vi "MainApp.vi"() -> ()   [LabVIEW 2018]
uses:
  TyDefApp/StatesApp.ctl
  TypeDefSERVER/PersonaFisica.ctl
  TypeDefSERVER/PersonaMoral.ctl
  TypeDefSERVER/ID_REQUEST.ctl
  <vilib>/httpClient/PUTBuffer.vi
  <vilib>/Utility/config.llb/Read Key (String).vi
  <vilib>/Utility/config.llb/Write Key (String).vi
  <vilib>/httpClient/LabVIEWHTTPClient.lvlib
  <vilib>/Utility/config.llb/NI_LVConfig.lvlib
panel:
  in  "MenuOpciones":enum32{"MenuPrincipal", "MenuCreditoPyme"}(tab)
  in  "SolicitudesRecientes_btn":bool
  in  "CreditoPyme_btn":bool
  out "CreditoPyme_select":bool
  out "SolicitudesRecientes_select":bool
  in  "PersonaFisica_btn":bool
  in  "PersonaMoral_btn":bool
  out "PersonaMoral_select":bool
  out "PersonaFisica_select":bool
  in  "PaginasPrincipales":T1(tab)
  in  "NoTengoCuenta_btn":bool
  in  "SoyCliente_btn":bool
  in  "SolicitudesRecientes_table":i32(listbox)
  in  "FinalizarSolicitud_btn":bool
  in  "IrADatosEspecificos_btn":bool caption="Siguiente:"
  in  "inicio_btn":bool
  in  "MenuPersonaFisica_Moral":T2(tab)
  in  "¿Para que es el credito?":string
  in  "Años de tu negocio:":i32
  in  "Sector de tu negocio:":string
  in  "Correo:":string
  in  "Celular (10 digitos):":string
  in  "RFC con homoclave:":string
  in  "Apellido paterno:":string
  in  "Apellido materno:":string
  in  "Nombre:":string
  in  "Correo_Moral":string caption="Correo:"
  in  "Celular_Moral":string caption="Celular (10 digitos):"
  in  "ApellidoPaterno_Moral":string caption="Apellido paterno:"
  in  "ApellidoMaterno_Moral":string caption="Apellido materno:"
  in  "Nombre_Moral":string caption="Nombre:"
  in  "Moral1_btn":bool
  in  "RazonSocial":string caption="Razon social:"
  in  "RFC_Moral":string caption="RFC con homoclave:"
  in  "SectorDeNegocio_Moral2":string caption="Sector de tu negocio:"
  in  "AñosDenegocio_Moral2":i32 caption="Años de tu negocio:"
  in  "ParaQueCredito_Moral2":string caption="¿Para que es el credito?"
  in  "Moral2_btn":bool caption="Back Tool"
  in  "Garantia, patrimonio (valor):":dbl format="$%#_g"
  in  "Numero de empleados:":i32
  in  "Numero de sucursales:":i32
  in  "Regimen que tributa:":string
  in  "Años de antiguedad de la empresa:":i32
  in  "Flujo de efectivo mensual:":dbl format="$%#_g"
  in  "Utilidad neta:":dbl format="$%#_g"
  in  "Capital social:":dbl format="$%#_g"
  in  "Importe Total:":dbl format="$%#_g"
  # "Solicita tu credito Pyme aqui."
  # "Solicitud de credito para cliente BBVA"
  # "Datos del presentante legal:"
  # "Datos del negocio"
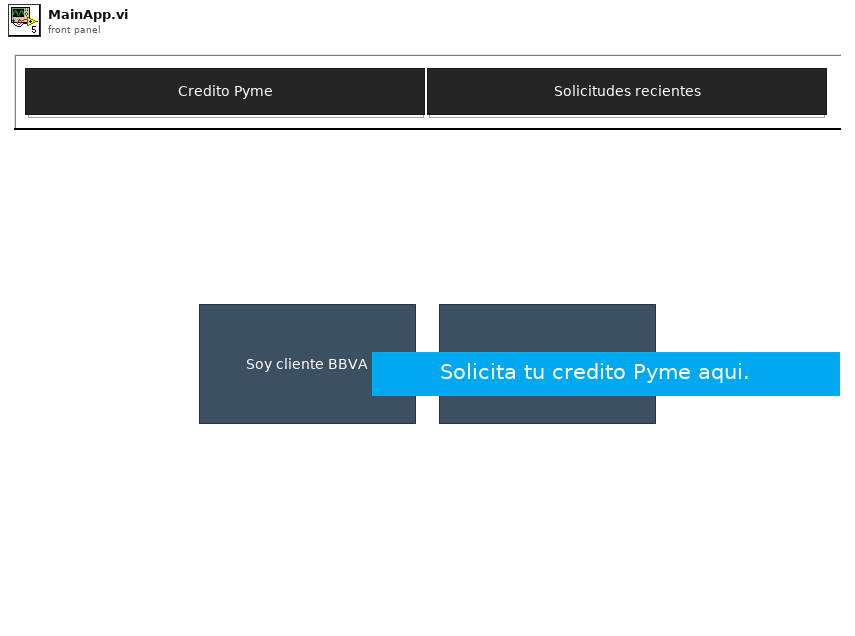
[diagram p1: front panel]
types:
  T1 = enum32{"CreditoPyme", "SolicitudesRecientes", "PersonaFisica", "PersonaMoral", "None", "DatosEspecificos"}
  T2 = enum32{"PersonaFisica", "PersonaMoral1", "PersonaMoral 2", "DatosEspecificos"}
  T3 = enum16{"init", "standBy", "goToCreditoPyme", "goToSolicitudesRecientes", "goToPersonaFisica", "goToPersonaMoral1", "goToPersonaMoral2", "goToDatosEspecificos", "ClearEntrys", "DeleteHistorial", "ShowSolicitudAceptada", "ShowSolicitudCancelada", "RegisterSolicitudToCheck", "CloseApp"}
  T4 = typedef "StatesApp.ctl" = cluster{"Machine":enum16{"StateMachine", "Queues"}, "States":enum16{"init", "standBy", "goToCreditoPyme", "goToSolicitudesRecientes", "goToPersonaFisica", "goToPersonaMoral1", "goToPersonaMoral2", "goToDatosEspecificos", "ClearEntrys", "DeleteHistorial", "ShowSolicitudAceptada", "ShowSolicitudCancelada", "RegisterSolicitudToCheck", "CloseApp", "goToPersonaMoral", "CheckIsClient"}, "URL":string, "TipoPersona":string, "EsCliente?":bool, "ID_CARD":string}
  T5 = enum32{"Invalid", "Standard", "Closed", "Hidden", "Minimized", "Maximized"}
  T6 = typedef "NI_LVConfig.lvlib/Config Data RefNum.ctl" = refnum<k1>
  T7 = typedef "PersonaFisica.ctl" = cluster{"Sector de tu negocio":string, "Para que es el credito":string, "Correo":string, "RFC con homoclave":string, "Nombre":string, "Celular":string, "Apellido materno":string, "Apellido paterno":string, "Años de tu negocio:":i32, "Numero de tarjeta":string, "EsCliente?":bool, "Importe Total":dbl, "Capital social":dbl, "Flujo de efectivo mensual":dbl, "Utilidad neta":dbl, "Garantia, patrimonio (valor):":dbl, "Numero de sucursales":i32, "Numero de empleados":i32, "Años de antiguedad de la empresa":i32, "Regimen que tributa":string, "Confirmado?":bool, "TipoPersona":string}
  T8 = typedef "PersonaMoral.ctl" = cluster{"Sector del negocio":string, "Para que el credito":string, "RFC":string, "RazonSocial":string, "Apellido paterno":string, "Nombre":string, "Correo":string, "Apellido materno":string, "Celular":string, "AñosDenegocio":i32, "Numero de tarjeta":string, "EsCliente?":bool, "Importe Total":dbl, "Capital social":dbl, "Flujo de efectivo mensual":dbl, "Utilidad neta":dbl, "Garantia, patrimonio (valor):":dbl, "Numero de sucursales":i32, "Numero de empleados":i32, "Años de antiguedad de la empresa":i32, "Regimen que tributa":string, "Confirmado?":bool, "TipoPersona":string}
  T9 = enum16{"CreditoPyme", "SolicitudeRecientes", "PersonaFisica", "PersonaMoral"}
  T10 = enum16{"init", "standBy", "goToCreditoPyme", "goToSolicitudesRecientes", "goToPersonaFisica", "goToPersonaMoral1", "goToPersonaMoral2", "goToDatosEspecificos", "ClearEntrys", "DeleteHistorial", "ShowSolicitudAceptada", "ShowSolicitudCancelada", "RegisterSolicitudToCheck", "CloseApp", "goToPersonaMoral"}
  T11 = enum32{"PersonaFisica", "PersonaMoral1", "PersonaMoral 2"}
  T12 = enum16{"init", "standBy", "goToCreditoPyme", "goToSolicitudesRecientes", "goToPersonaFisica", "goToPersonaMoral1", "goToPersonaMoral2", "goToDatosEspecificos", "ClearEntrys", "DeleteHistorial", "ShowSolicitudAceptada", "ShowSolicitudCancelada", "RegisterSolicitudToCheck", "CloseApp", "goToPersonaMoral", "CheckIsClient"}
  T13 = typedef "ID_REQUEST.ctl" = cluster{"ID":i32[]}
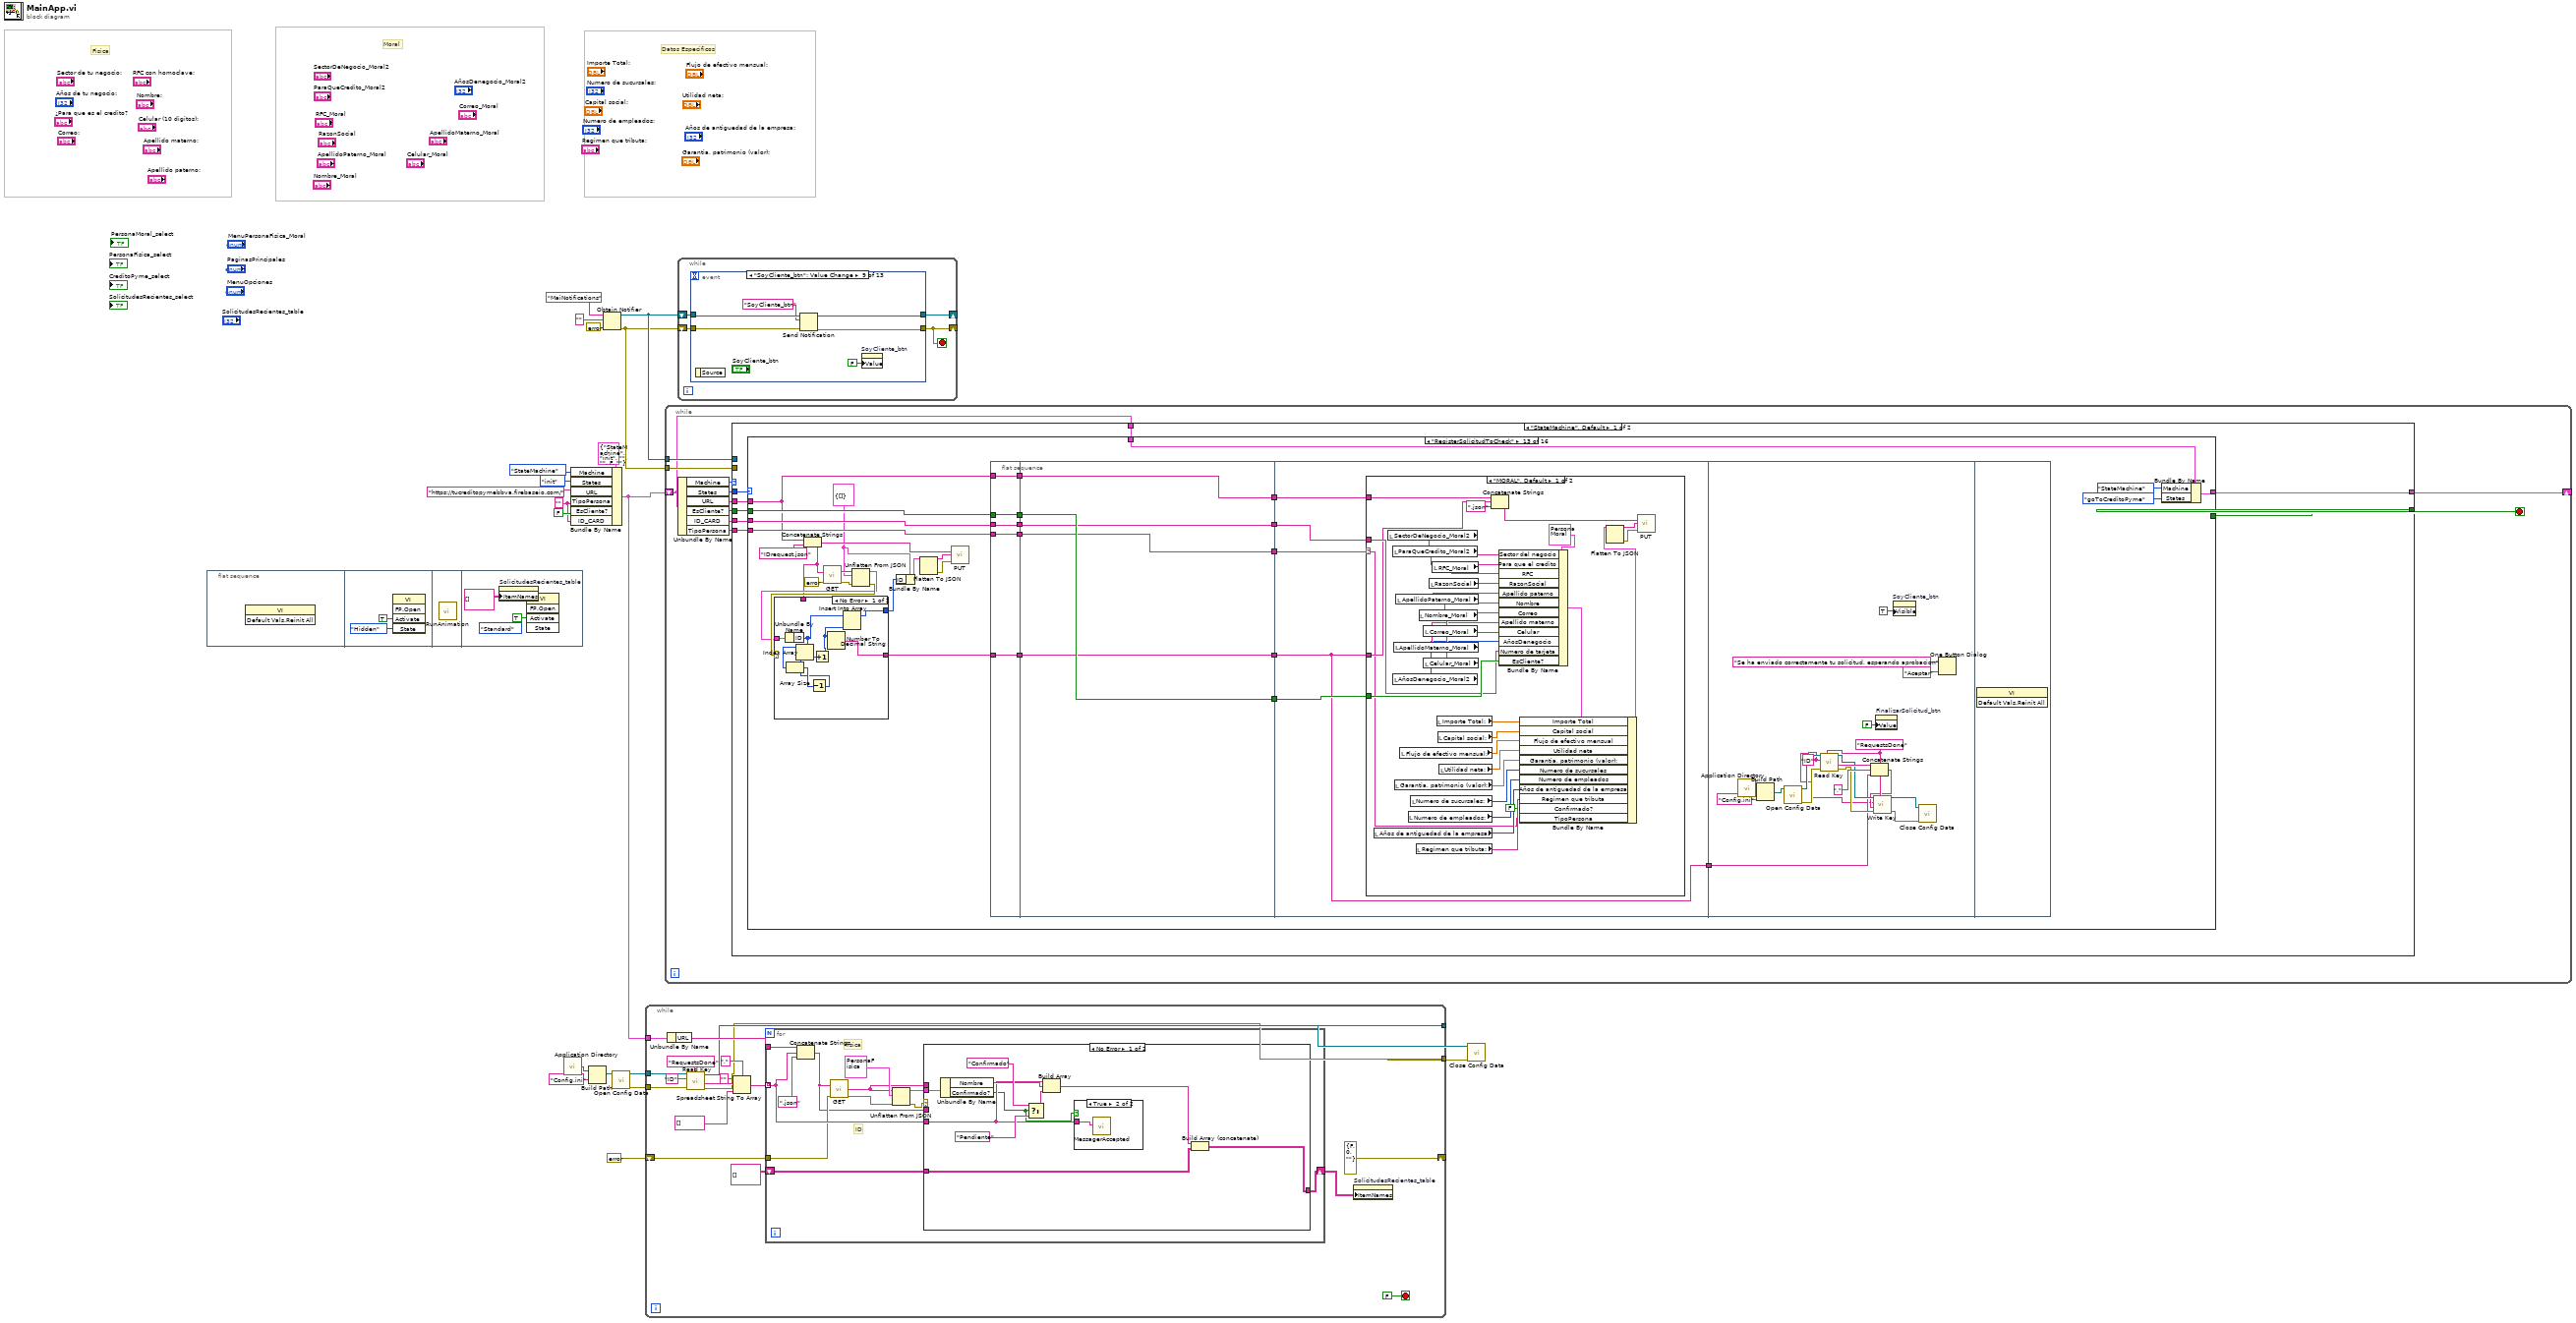
[diagram p0: block diagram]
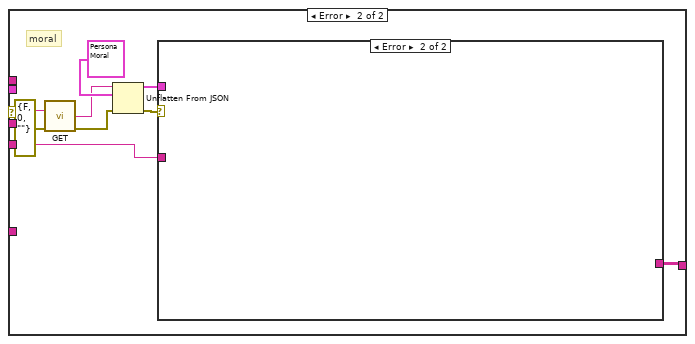
[diagram p3: hidden frame]
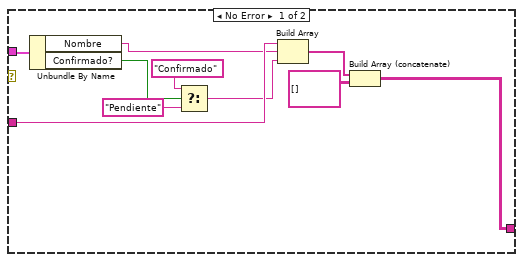
[diagram p4: hidden frame]
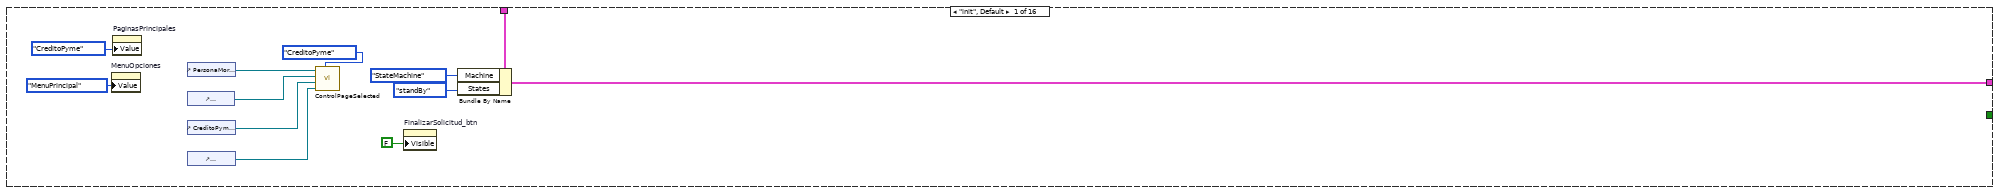
[diagram p5: hidden frame]
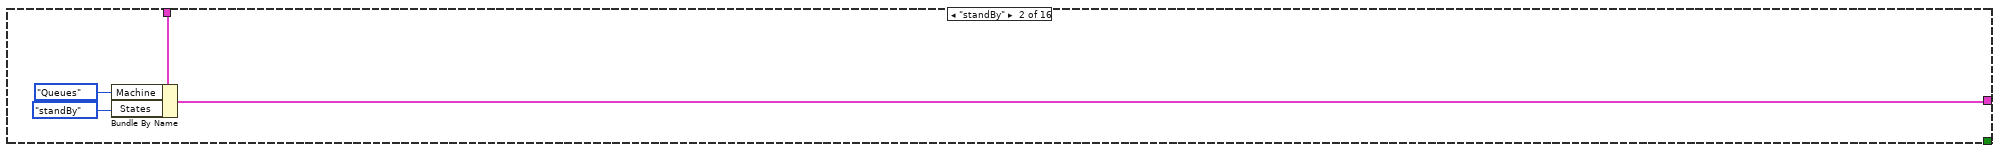
[diagram p6: hidden frame]
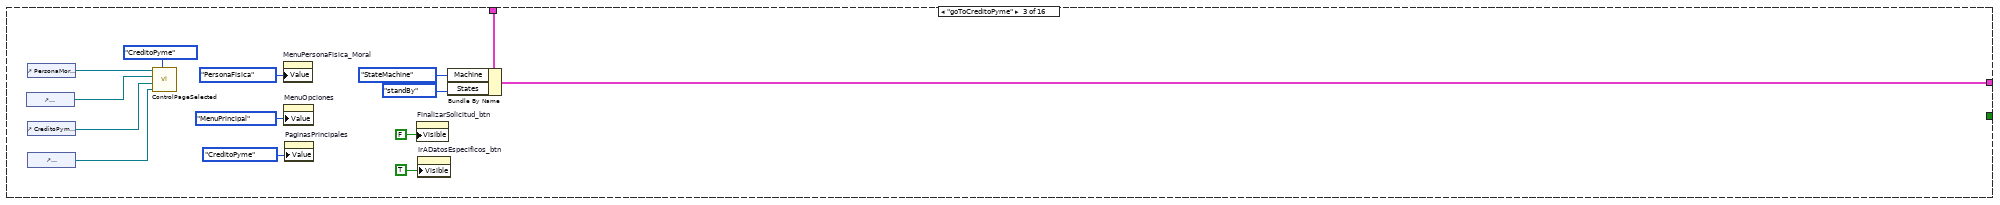
[diagram p7: hidden frame]
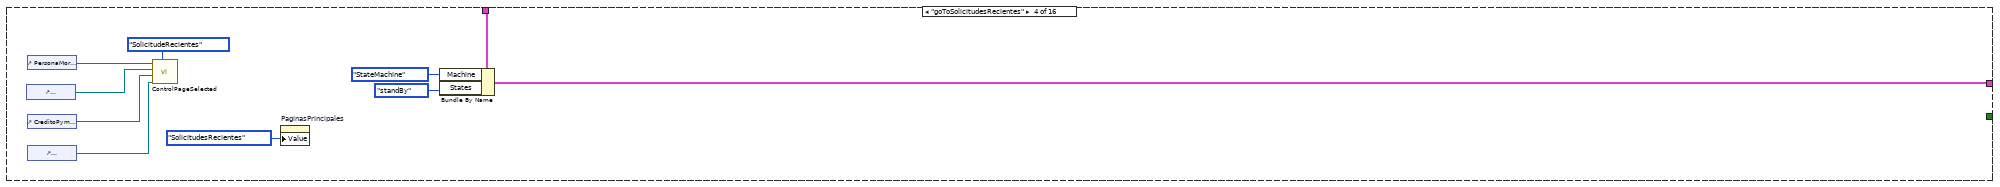
[diagram p8: hidden frame]
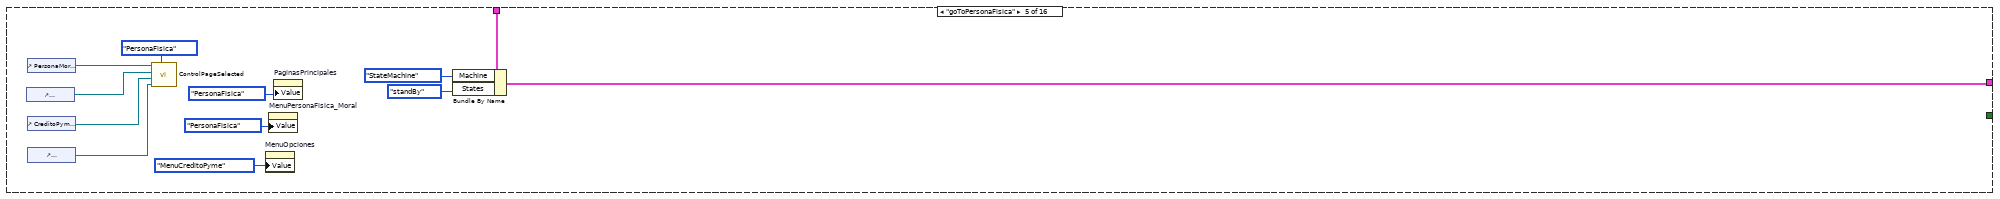
[diagram p9: hidden frame]
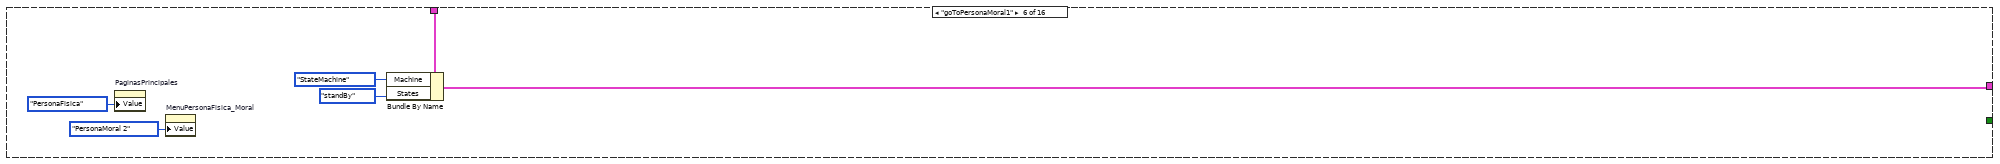
[diagram p10: hidden frame]
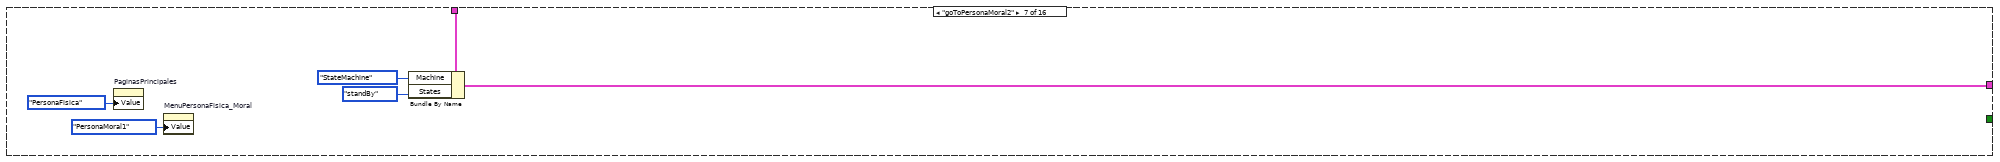
[diagram p11: hidden frame]
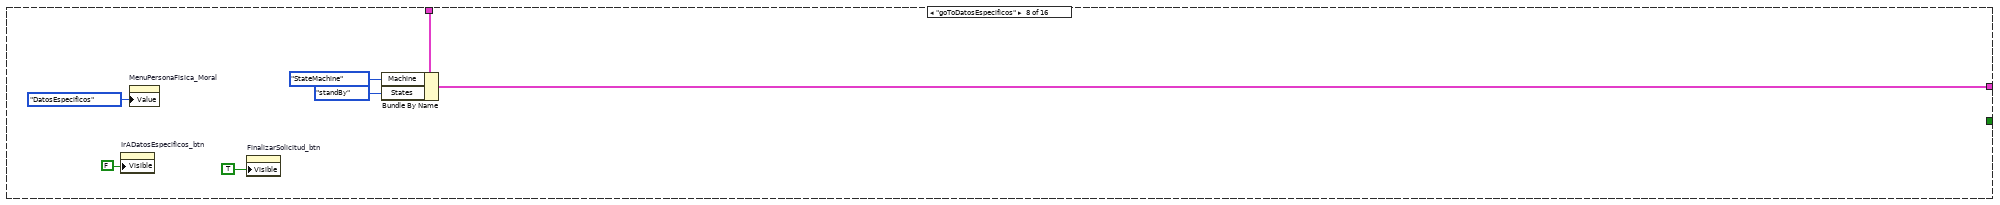
[diagram p12: hidden frame]
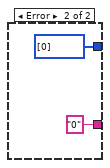
[diagram p17: hidden frame]
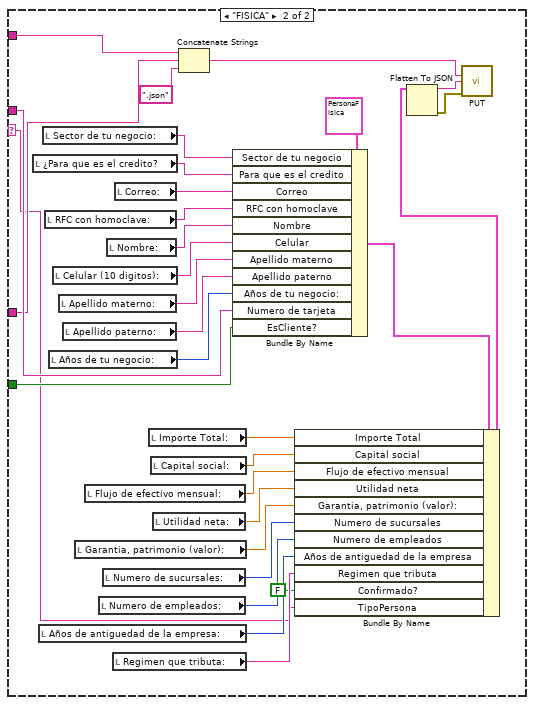
[diagram p18: hidden frame]
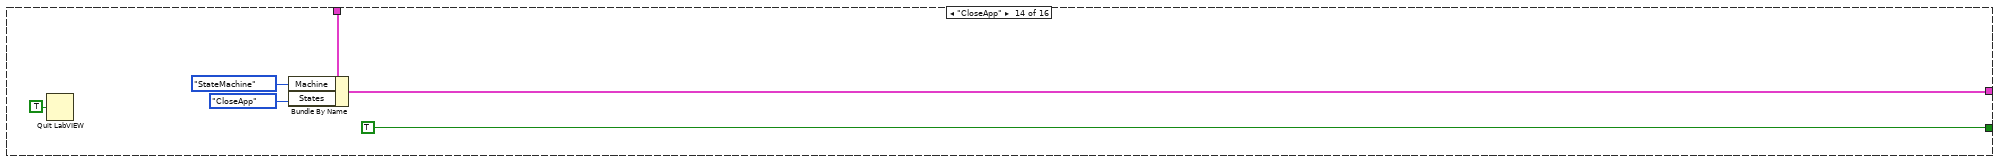
[diagram p19: hidden frame]
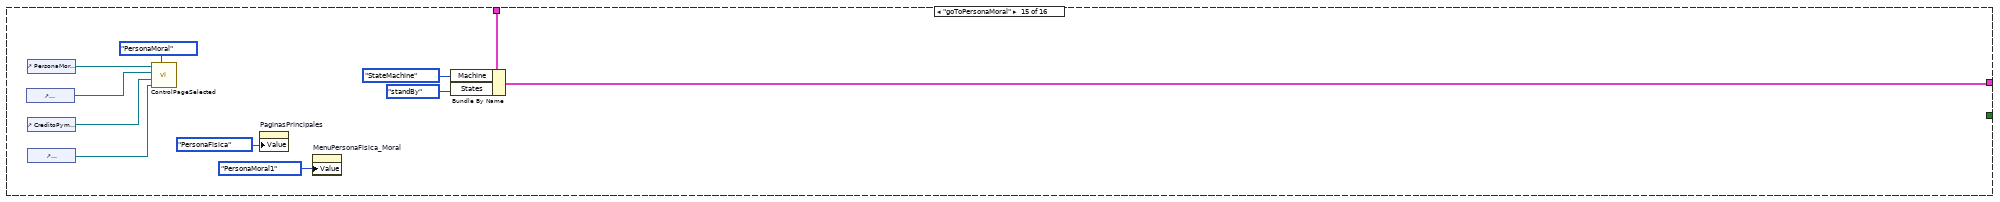
[diagram p20: hidden frame]
diagram:
  w10 = "" ("TipoPersona")
  # "Datos Especificos"
  # "Moral"
  # "Fisica"
  n1 = flat-sequence {
    frame #0 {
      n2 = invoke class="VI" method="Default Vals.Reinit All"() -> ()  [unwired: 3 in, 3 out]
    }
    frame #1 {
      n3 = invoke class="VI" method="FP.Open"("Activate"=TRUE ("Activate?"), "State"=T5."Hidden") -> ()  [unwired: 3 in, 5 out]
    }
    frame #2 {
      n4 = call "RunAnimation.vi"() -> ()  [unwired: 12 in]
    }
    frame #3 {
      (unwired) T5."Standard" ("State")
      n5 = property on="SolicitudesRecientes_table" class="MCListbox (strict)"("ItemNames"=string[][] [] ("Item Names")) -> ()  [unwired: 2 in, 2 out]
      n6 = invoke class="VI" method="FP.Open"("Activate"=TRUE ("Activate?")) -> ()  [unwired: 4 in, 5 out]
    }
  }
  n7 = call <vilib>:"Application Directory.vi"() -> ("Application Directory"=w7:path)
  n8 = Bundle By Name(cluster=T4 {"Machine"=enum."StateMachine", "States"=enum."init", "URL"="", "TipoPersona"="", "EsCliente?"=FALSE, "ID_CARD"=""} ("Cluster"), "Machine"=enum16{"StateMachine", "Queues"}."StateMachine", "States"=T3."init", "URL"="https://tucreditopymebbva.firebaseio.com/", "TipoPersona"=w10, "EsCliente?"=FALSE, "ID_CARD"=w10) -> (w4:T4)
  n9 = Build Path(base path=w7, name or relative path="Config.ini") -> (appended path=w5:path)
  n10 = Obtain Notifier(name (unnamed)="MaiNotifications", notification data type="", error in (no error)=errorcluster {"status"=FALSE, "code"=0, "source"=""}) -> (notifier out=w16:refnum<notifier>, error out=w15:errorcluster)  [unwired: 1 in, 1 out]
  n11 = call <vilib>:"Open Config Data.vi"("configuration file path"=w5) -> ("error out"=w8:errorcluster, "refnum"=w9:T6)  [unwired: 8 in, 1 out]
  n12 = while {
    tunnel: w9 -> [w41]
    tunnel: w8 -> [w40]
    tunnel: w4 -> [w33]
    tunnel: [w31] -> w3
    tunnel: [w30] -> w2
    shift-right: [errorcluster {"status"=FALSE, "code"=0, "source"=""} ("error in (no error)")] -> _
    shift-left: errorcluster {"status"=FALSE, "code"=0, "source"=""} ("error in (no error)") -> [w28]
    stop <- FALSE stop-if-true
    n13 = Unbundle By Name(w33) -> ("URL"=w32:string)
    n14 = call-poly <vilib>:"Read Key.vi"("section"="RequestsDone", "error in (no error)"=w40, "key"="ID", "refnum"=w41) -> ("error out"=w30:errorcluster, "value"=w37:string, "refnum out"=w31:T6)  [unwired: 4 in, 1 out]
    n15 = Spreadsheet String To Array(delimiter (Tab)=",", format string="", spreadsheet string=w37, array type (2D Dbl)=string[] []) -> (array=w34:string[])
    n16 = for {
      tunnel: w34 -> [w48] mode=indexing
      tunnel: w32 -> [w54]
      tunnel: w28 -> [w46]
      shift-right: [w44] -> w26
      shift-left: string[][] [] -> [w43]
      # "ID"
      # "fisica"
      n17 = Concatenate Strings(w54, w48, ".json" ("string")) -> (w45:string)
      n18 = call <vilib>:"GET.vi"("url"=w45, "error in (no error)"=w46) -> ("body"=w47:string, "error out"=w52:errorcluster)  [unwired: 10 in, 2 out]
      n19 = Unflatten From JSON(JSON string=w47, type and defaults=T7 {"Sector de tu negocio"="", "Para que es el credito"="", "Correo"="", "RFC con homoclave"="", "Nombre"="", "Celular"="", "Apellido materno"="", "Apellido paterno"="", "Años de tu negocio:"=0, "Numero de tarjeta"="", "EsCliente?"=FALSE, "Importe Total"=0.0, "Capital social"=0.0, "Flujo de efectivo mensual"=0.0, "Utilidad neta"=0.0, "Garantia, patrimonio (valor):"=0.0, "Numero de sucursales"=0, "Numero de empleados"=0, "Años de antiguedad de la empresa"=0, "Regimen que tributa"="", "Confirmado?"=FALSE, "TipoPersona"=""} ("Cluster"), error in (no error)=w52) -> (value=w49:T7, error out=w50:errorcluster)  [unwired: 4 in]
      n20 = case shown="No Error" w50 {
        tunnel: w49 -> [w64 _]
        tunnel: w47 -> [_ _]
        tunnel: w48 -> [w57 w71]
        tunnel: [w59 w70] -> w44
        tunnel: w45 -> [_ w67]
        tunnel: w43 -> [w58 _]
        frame No Error {
          n21 = Unbundle By Name(w64) -> ("Nombre"=w61:string, "Confirmado?"=w55:bool)
          n22 = Select(t="Confirmado", s=w55, f="Pendiente") -> (s? t:f=w56:string)
          n23 = Build Array(w57, w61, w56) -> (w60:string[])
          n24 = case shown="True" w55 {
            tunnel: w57 -> [_ w65]
            frame False {
            }
            frame True {
              n25 = call "MessagerAccepted.vi"("id"=w65) -> ()  [unwired: 11 in]
            }
          }
          n26 = Build Array (concatenate)(w60, w58) -> (w59:string[][])
        }
        frame Error {
          # "moral"
          n27 = call <vilib>:"GET.vi"("url"=w67, "error in (no error)"=errorcluster {"status"=FALSE, "code"=0, "source"=""}) -> ("body"=w68:string, "error out"=w69:errorcluster)  [unwired: 10 in, 2 out]
          n28 = Unflatten From JSON(JSON string=w68, type and defaults=T8 {"Sector del negocio"="", "Para que el credito"="", "RFC"="", "RazonSocial"="", "Apellido paterno"="", "Nombre"="", "Correo"="", "Apellido materno"="", "Celular"="", "AñosDenegocio"=0, "Numero de tarjeta"="", "EsCliente?"=FALSE, "Importe Total"=0.0, "Capital social"=0.0, "Flujo de efectivo mensual"=0.0, "Utilidad neta"=0.0, "Garantia, patrimonio (valor):"=0.0, "Numero de sucursales"=0, "Numero de empleados"=0, "Años de antiguedad de la empresa"=0, "Regimen que tributa"="", "Confirmado?"=FALSE, "TipoPersona"=""} ("Cluster"), error in (no error)=w69) -> (value=w72:T8, error out=w73:errorcluster)  [unwired: 4 in]
          n29 = case shown="Error" w73 {
            tunnel: w72 -> [w84 _]
            tunnel: w71 -> [w80 _]
            tunnel: [w75 _] -> w70
            frame No Error {
              n30 = Unbundle By Name(w84) -> ("Nombre"=w79:string, "Confirmado?"=w83:bool)
              n31 = Select(t="Confirmado", s=w83, f="Pendiente") -> (s? t:f=w78:string)
              n32 = Build Array(w80, w79, w78) -> (w77:string[])
              n33 = Build Array (concatenate)(w77, string[][] [] ("element")) -> (w75:string[][])
            }
            frame Error {
            }
          }
        }
      }
    }
    n34 = property on="SolicitudesRecientes_table" class="MCListbox (strict)"("ItemNames"=w26) -> ()  [unwired: 2 in, 2 out]
  }
  n35 = while {
    shift-right: [w89] -> _
    shift-left: w4 -> [w90]
    tunnel: w16 -> [w92]
    tunnel: w15 -> [w91]
    stop <- w88 stop-if-true
    n36 = Unbundle By Name(w90) -> ("Machine"=w95:enum16{"StateMachine", "Queues"}, "States"=w94:T12, "URL"=w93:string, "EsCliente?"=w87:bool, "ID_CARD"=w86:string, "TipoPersona"=w85:string)
    n37 = case shown="\"StateMachine\", Default" w95 {
      tunnel: w94 -> [w103 _]
      tunnel: w93 -> [w102 _]
      tunnel: w92 -> [_ w347]
      tunnel: w91 -> [_ w346]
      tunnel: w90 -> [w98 w344]
      tunnel: [w101 w343] -> w89
      tunnel: [w100 _] -> w88
      tunnel: w87 -> [w99 _]
      tunnel: w86 -> [w97 _]
      tunnel: w85 -> [w96 _]
      frame "StateMachine", Default {
        n38 = case shown="\"RegisterSolicitudToCheck\"" w103 {
          tunnel: w102 -> [_ _ _ _ _ _ _ _ _ _ _ _ w191 _ _ _]
          tunnel: w98 -> [w113 w119 w133 w141 w153 w159 w165 w174 _ _ _ _ w206 w317 w328 w333]
          tunnel: [w112 w118 w132 w140 w152 w158 w164 w173 _ _ _ _ w205 w316 w327 w332] -> w101
          tunnel: [_ _ _ _ _ _ _ _ _ _ _ _ _ TRUE _ _] -> w100
          tunnel: w99 -> [_ _ _ _ _ _ _ _ _ _ _ _ w201 _ _ w334]
          tunnel: w97 -> [_ _ _ _ _ _ _ _ _ _ _ _ w200 _ _ _]
          tunnel: w96 -> [_ _ _ _ _ _ _ _ _ _ _ _ w202 _ _ _]
          frame "init", Default {
            n39 = property on="MenuOpciones" class="TabCtl (strict)"("Value"=enum32{"MenuPrincipal", "MenuCreditoPyme"}."MenuPrincipal" ("MenuOpciones")) -> ()  [unwired: 2 in, 2 out]
            n40 = property on="PaginasPrincipales" class="TabCtl (strict)"("Value"=T1."CreditoPyme" ("PaginasPrincipales")) -> ()  [unwired: 2 in, 2 out]
            n41 = control-ref of="PersonaFisica_select"() -> (w109:refnum<vi>)
            n42 = control-ref of="PersonaMoral_select"() -> (w110:refnum<vi>)
            n43 = control-ref of="CreditoPyme_select"() -> (w108:refnum<vi>)
            n44 = control-ref of="SolicitudesRecientes_select"() -> (w107:refnum<vi>)
            n45 = call "ControlPageSelected.vi"("PageSelected"=T9."CreditoPyme", "SolicitudesRecientes"=w107, "CreditoPyme"=w108, "PersonaFisica"=w109, "PersonaMoral"=w110) -> ()  [unwired: 7 in]
            n46 = property on="FinalizarSolicitud_btn" class="Bool (strict)"("Visible"=FALSE) -> ()  [unwired: 2 in, 2 out]
            n47 = Bundle By Name(cluster=w113, "Machine"=enum16{"StateMachine", "Queues"}."StateMachine", "States"=T3."standBy") -> (w112:T4)
          }
          frame "standBy" {
            n48 = Bundle By Name(cluster=w119, "Machine"=enum16{"StateMachine", "Queues"}."Queues", "States"=T3."standBy") -> (w118:T4)
          }
          frame "goToCreditoPyme" {
            n49 = control-ref of="PersonaFisica_select"() -> (w128:refnum<vi>)
            n50 = control-ref of="PersonaMoral_select"() -> (w129:refnum<vi>)
            n51 = control-ref of="CreditoPyme_select"() -> (w127:refnum<vi>)
            n52 = control-ref of="SolicitudesRecientes_select"() -> (w126:refnum<vi>)
            n53 = call "ControlPageSelected.vi"("PageSelected"=T9."CreditoPyme", "SolicitudesRecientes"=w126, "CreditoPyme"=w127, "PersonaFisica"=w128, "PersonaMoral"=w129) -> ()  [unwired: 7 in]
            n54 = property on="MenuPersonaFisica_Moral" class="TabCtl (strict)"("Value"=T2."PersonaFisica" ("MenuPersonaFisica_Moral")) -> ()  [unwired: 2 in, 2 out]
            n55 = property on="MenuOpciones" class="TabCtl (strict)"("Value"=enum32{"MenuPrincipal", "MenuCreditoPyme"}."MenuPrincipal" ("MenuOpciones")) -> ()  [unwired: 2 in, 2 out]
            n56 = property on="PaginasPrincipales" class="TabCtl (strict)"("Value"=T1."CreditoPyme" ("PaginasPrincipales")) -> ()  [unwired: 2 in, 2 out]
            n57 = property on="FinalizarSolicitud_btn" class="Bool (strict)"("Visible"=FALSE ("FinalizarSolicitud_btn")) -> ()  [unwired: 2 in, 2 out]
            n58 = property on="IrADatosEspecificos_btn" class="Bool (strict)"("Visible"=TRUE) -> ()  [unwired: 2 in, 2 out]
            n59 = Bundle By Name(cluster=w133, "Machine"=enum16{"StateMachine", "Queues"}."StateMachine", "States"=T10."standBy") -> (w132:T4)
          }
          frame "goToSolicitudesRecientes" {
            n60 = control-ref of="PersonaFisica_select"() -> (w138:refnum<vi>)
            n61 = control-ref of="PersonaMoral_select"() -> (w139:refnum<vi>)
            n62 = control-ref of="CreditoPyme_select"() -> (w137:refnum<vi>)
            n63 = control-ref of="SolicitudesRecientes_select"() -> (w136:refnum<vi>)
            n64 = call "ControlPageSelected.vi"("PageSelected"=T9."SolicitudeRecientes", "SolicitudesRecientes"=w136, "CreditoPyme"=w137, "PersonaFisica"=w138, "PersonaMoral"=w139) -> ()  [unwired: 7 in]
            n65 = property on="PaginasPrincipales" class="TabCtl (strict)"("Value"=T1."SolicitudesRecientes" ("PaginasPrincipales")) -> ()  [unwired: 2 in, 2 out]
            n66 = Bundle By Name(cluster=w141, "Machine"=enum16{"StateMachine", "Queues"}."StateMachine", "States"=T10."standBy") -> (w140:T4)
          }
          frame "goToPersonaFisica" {
            n67 = control-ref of="PersonaFisica_select"() -> (w150:refnum<vi>)
            n68 = control-ref of="PersonaMoral_select"() -> (w151:refnum<vi>)
            n69 = control-ref of="CreditoPyme_select"() -> (w149:refnum<vi>)
            n70 = control-ref of="SolicitudesRecientes_select"() -> (w148:refnum<vi>)
            n71 = call "ControlPageSelected.vi"("PageSelected"=T9."PersonaFisica", "SolicitudesRecientes"=w148, "CreditoPyme"=w149, "PersonaFisica"=w150, "PersonaMoral"=w151) -> ()  [unwired: 7 in]
            n72 = property on="MenuOpciones" class="TabCtl (strict)"("Value"=enum32{"MenuPrincipal", "MenuCreditoPyme"}."MenuCreditoPyme" ("MenuOpciones")) -> ()  [unwired: 2 in, 2 out]
            n73 = property on="MenuPersonaFisica_Moral" class="TabCtl (strict)"("Value"=T11."PersonaFisica" ("MenuPersonaFisica_Moral")) -> ()  [unwired: 2 in, 2 out]
            n74 = property on="PaginasPrincipales" class="TabCtl (strict)"("Value"=T1."PersonaFisica" ("PaginasPrincipales")) -> ()  [unwired: 2 in, 2 out]
            n75 = Bundle By Name(cluster=w153, "Machine"=enum16{"StateMachine", "Queues"}."StateMachine", "States"=T10."standBy") -> (w152:T4)
          }
          frame "goToPersonaMoral1" {
            n76 = property on="PaginasPrincipales" class="TabCtl (strict)"("Value"=T1."PersonaFisica" ("PaginasPrincipales")) -> ()  [unwired: 2 in, 2 out]
            n77 = property on="MenuPersonaFisica_Moral" class="TabCtl (strict)"("Value"=T11."PersonaMoral 2" ("MenuPersonaFisica_Moral")) -> ()  [unwired: 2 in, 2 out]
            n78 = Bundle By Name(cluster=w159, "Machine"=enum16{"StateMachine", "Queues"}."StateMachine", "States"=T10."standBy") -> (w158:T4)
          }
          frame "goToPersonaMoral2" {
            n79 = property on="PaginasPrincipales" class="TabCtl (strict)"("Value"=T1."PersonaFisica" ("PaginasPrincipales")) -> ()  [unwired: 2 in, 2 out]
            n80 = property on="MenuPersonaFisica_Moral" class="TabCtl (strict)"("Value"=T11."PersonaMoral1" ("MenuPersonaFisica_Moral")) -> ()  [unwired: 2 in, 2 out]
            n81 = Bundle By Name(cluster=w165, "Machine"=enum16{"StateMachine", "Queues"}."StateMachine", "States"=T10."standBy") -> (w164:T4)
          }
          frame "goToDatosEspecificos" {
            n82 = property on="IrADatosEspecificos_btn" class="Bool (strict)"("Visible"=FALSE) -> ()  [unwired: 2 in, 2 out]
            n83 = property on="MenuPersonaFisica_Moral" class="TabCtl (strict)"("Value"=T2."DatosEspecificos" ("MenuPersonaFisica_Moral")) -> ()  [unwired: 2 in, 2 out]
            n84 = property on="FinalizarSolicitud_btn" class="Bool (strict)"("Visible"=TRUE ("FinalizarSolicitud_btn")) -> ()  [unwired: 2 in, 2 out]
            n85 = Bundle By Name(cluster=w174, "Machine"=enum16{"StateMachine", "Queues"}."StateMachine", "States"=T10."standBy") -> (w173:T4)
          }
          frame "ClearEntrys" {
          }
          frame "DeleteHistorial" {
          }
          frame "ShowSolicitudAceptada" {
          }
          frame "ShowSolicitudCancelada" {
          }
          frame "RegisterSolicitudToCheck" {
            w186 = T13 {"ID"=[]} ("Cluster")
            n86 = Concatenate Strings(w191, "IDrequest.json" ("string")) -> (w187:string)
            n87 = call <vilib>:"GET.vi"("url"=w187, "error in (no error)"=errorcluster {"status"=FALSE, "code"=0, "source"=""}) -> ("body"=w194:string, "error out"=w193:errorcluster)  [unwired: 10 in, 2 out]
            n88 = Unflatten From JSON(JSON string=w194, type and defaults=w186, error in (no error)=w193) -> (value=w188:T13, error out=w189:errorcluster)  [unwired: 4 in]
            n89 = case shown="No Error" w189 {
              tunnel: w188 -> [w214 _]
              tunnel: [w207 "0"] -> w181
              tunnel: w187 -> [_ _]
              tunnel: [w213 i32[] [0]] -> w185
              frame No Error {
                n90 = Unbundle By Name(w214) -> ("ID"=w212:i32[])
                n91 = Array Size(array=w212) -> (size(s)=w211:i32)
                n92 = Decrement(x=w211) -> (x-1=w210:i32)
                n93 = Index Array(array=w212, index=w210) -> (element=w209:i32)
                n94 = Increment(x=w209) -> (x+1=w208:i32)
                n95 = Number To Decimal String(number=w208) -> (decimal integer string=w207:string)  [unwired: 1 in]
                n96 = Insert Into Array(array=w212, new element=w208) -> (w213:i32[])  [unwired: 1 in]
              }
              frame Error {
              }
            }
            n97 = Bundle By Name(cluster=w186, "ID"=w185) -> (w184:T13)
            n98 = Flatten To JSON(anything=w184) -> (JSON string=w183:string, 11:w182:errorcluster)  [unwired: 2 in]
            n99 = call-poly <vilib>:"PUT.vi"("url"=w187, "buffer"=w183, "error in (no error)"=w182) -> ()  [unwired: 9 in, 4 out]
            n100 = flat-sequence {
              tunnel: w191 -> [w218]
              tunnel: w200 -> [w219]
              tunnel: w201 -> [w220]
              tunnel: w202 -> [w221]
              tunnel: [w221] -> w198
              tunnel: [w220] -> w197
              tunnel: [w219] -> w196
              tunnel: [w218] -> w195
              tunnel: w181 -> [w217]
              tunnel: [w217] -> w177
              tunnel: [w222] -> w199
              tunnel: w198 -> [w222]
              tunnel: w197 -> [w226]
              tunnel: w196 -> [w225]
              tunnel: w195 -> [w224]
              tunnel: [w226] -> w180
              tunnel: [w225] -> w179
              tunnel: [w224] -> w178
              tunnel: w177 -> [w223]
              tunnel: [w223] -> w176
              tunnel: w199 -> [w228]
              tunnel: w180 -> [w231]
              tunnel: w179 -> [w230]
              tunnel: w178 -> [w229]
              tunnel: w176 -> [w227]
              tunnel: [w227] -> w175
              tunnel: w175 -> [w296]
              frame #0 {
              }
              frame #1 {
              }
              frame #2 {
                n101 = case shown="\"MORAL\", Default" w228 {
                  selector: w228 -> [w233 w265]
                  tunnel: w231 -> [w252 w284]
                  tunnel: w230 -> [w251 w283]
                  tunnel: w229 -> [w232 w264]
                  tunnel: w227 -> [w250 w282]
                  frame "MORAL", Default {
                    n102 = local read "Años de antiguedad de la empresa:"() -> (w245:i32)
                    n103 = local read "SectorDeNegocio_Moral2"() -> (w262:string)
                    n104 = local read "ParaQueCredito_Moral2"() -> (w261:string)
                    n105 = local read "AñosDenegocio_Moral2"() -> (w253:i32)
                    n106 = local read "ApellidoMaterno_Moral"() -> (w254:string)
                    n107 = local read "Garantia, patrimonio (valor):"() -> (w241:dbl)
                    n108 = local read "ApellidoPaterno_Moral"() -> (w258:string)
                    n109 = local read "Flujo de efectivo mensual:"() -> (w239:dbl)
                    n110 = local read "Numero de empleados:"() -> (w243:i32)
                    n111 = local read "Numero de sucursales:"() -> (w242:i32)
                    n112 = local read "Regimen que tributa:"() -> (w244:string)
                    n113 = local read "Nombre_Moral"() -> (w257:string)
                    n114 = local read "Correo_Moral"() -> (w256:string)
                    n115 = local read "Celular_Moral"() -> (w255:string)
                    n116 = local read "RazonSocial"() -> (w259:string)
                    n117 = local read "RFC_Moral"() -> (w260:string)
                    n118 = local read "Importe Total:"() -> (w237:dbl)
                    n119 = local read "Capital social:"() -> (w238:dbl)
                    n120 = local read "Utilidad neta:"() -> (w240:dbl)
                    n121 = Concatenate Strings(w232, w250, ".json" ("string")) -> (w247:string)
                    n122 = Bundle By Name(cluster=T8 {"Sector del negocio"="", "Para que el credito"="", "RFC"="", "RazonSocial"="", "Apellido paterno"="", "Nombre"="", "Correo"="", "Apellido materno"="", "Celular"="", "AñosDenegocio"=0, "Numero de tarjeta"="", "EsCliente?"=FALSE, "Importe Total"=0.0, "Capital social"=0.0, "Flujo de efectivo mensual"=0.0, "Utilidad neta"=0.0, "Garantia, patrimonio (valor):"=0.0, "Numero de sucursales"=0, "Numero de empleados"=0, "Años de antiguedad de la empresa"=0, "Regimen que tributa"="", "Confirmado?"=FALSE, "TipoPersona"=""} ("Cluster"), "Sector del negocio"=w262, "Para que el credito"=w261, "RFC"=w260, "RazonSocial"=w259, "Apellido paterno"=w258, "Nombre"=w257, "Correo"=w256, "Apellido materno"=w254, "Celular"=w255, "AñosDenegocio"=w253, "Numero de tarjeta"=w251, "EsCliente?"=w252) -> (w236:T8)
                    n123 = Bundle By Name(cluster=w236, "Importe Total"=w237, "Capital social"=w238, "Flujo de efectivo mensual"=w239, "Utilidad neta"=w240, "Garantia, patrimonio (valor):"=w241, "Numero de sucursales"=w242, "Numero de empleados"=w243, "Años de antiguedad de la empresa"=w245, "Regimen que tributa"=w244, "Confirmado?"=FALSE, "TipoPersona"=w233) -> (w235:T8)
                    n124 = Flatten To JSON(anything=w235) -> (JSON string=w246:string, 11:w248:errorcluster)  [unwired: 2 in]
                    n125 = call-poly <vilib>:"PUT.vi"("url"=w247, "buffer"=w246, "error in (no error)"=w248) -> ()  [unwired: 9 in, 4 out]
                  }
                  frame "FISICA" {
                    n126 = local read "¿Para que es el credito?"() -> (w292:string)
                    n127 = local read "Años de antiguedad de la empresa:"() -> (w277:i32)
                    n128 = local read "Sector de tu negocio:"() -> (w293:string)
                    n129 = local read "RFC con homoclave:"() -> (w290:string)
                    n130 = local read "Años de tu negocio:"() -> (w285:i32)
                    n131 = local read "Celular (10 digitos):"() -> (w288:string)
                    n132 = local read "Apellido materno:"() -> (w287:string)
                    n133 = local read "Apellido paterno:"() -> (w286:string)
                    n134 = local read "Garantia, patrimonio (valor):"() -> (w273:dbl)
                    n135 = local read "Flujo de efectivo mensual:"() -> (w271:dbl)
                    n136 = local read "Numero de empleados:"() -> (w275:i32)
                    n137 = local read "Numero de sucursales:"() -> (w274:i32)
                    n138 = local read "Nombre:"() -> (w289:string)
                    n139 = local read "Regimen que tributa:"() -> (w276:string)
                    n140 = local read "Correo:"() -> (w291:string)
                    n141 = local read "Importe Total:"() -> (w269:dbl)
                    n142 = local read "Capital social:"() -> (w270:dbl)
                    n143 = local read "Utilidad neta:"() -> (w272:dbl)
                    n144 = Concatenate Strings(w264, w282, ".json" ("string")) -> (w279:string)
                    n145 = Bundle By Name(cluster=T7 {"Sector de tu negocio"="", "Para que es el credito"="", "Correo"="", "RFC con homoclave"="", "Nombre"="", "Celular"="", "Apellido materno"="", "Apellido paterno"="", "Años de tu negocio:"=0, "Numero de tarjeta"="", "EsCliente?"=FALSE, "Importe Total"=0.0, "Capital social"=0.0, "Flujo de efectivo mensual"=0.0, "Utilidad neta"=0.0, "Garantia, patrimonio (valor):"=0.0, "Numero de sucursales"=0, "Numero de empleados"=0, "Años de antiguedad de la empresa"=0, "Regimen que tributa"="", "Confirmado?"=FALSE, "TipoPersona"=""} ("Cluster"), "Sector de tu negocio"=w293, "Para que es el credito"=w292, "Correo"=w291, "RFC con homoclave"=w290, "Nombre"=w289, "Celular"=w288, "Apellido materno"=w287, "Apellido paterno"=w286, "Años de tu negocio:"=w285, "Numero de tarjeta"=w283, "EsCliente?"=w284) -> (w268:T7)
                    n146 = Bundle By Name(cluster=w268, "Importe Total"=w269, "Capital social"=w270, "Flujo de efectivo mensual"=w271, "Utilidad neta"=w272, "Garantia, patrimonio (valor):"=w273, "Numero de sucursales"=w274, "Numero de empleados"=w275, "Años de antiguedad de la empresa"=w277, "Regimen que tributa"=w276, "Confirmado?"=FALSE, "TipoPersona"=w265) -> (w267:T7)
                    n147 = Flatten To JSON(anything=w267) -> (JSON string=w278:string, 11:w280:errorcluster)  [unwired: 2 in]
                    n148 = call-poly <vilib>:"PUT.vi"("url"=w279, "buffer"=w278, "error in (no error)"=w280) -> ()  [unwired: 9 in, 4 out]
                  }
                }
              }
              frame #3 {
                w295 = "ID" ("key")
                w303 = "RequestsDone" ("section")
                n149 = call <vilib>:"Application Directory.vi"() -> ("Application Directory"=w311:path)
                n150 = Build Path(base path=w311, name or relative path="Config.ini") -> (appended path=w309:path)
                n151 = call <vilib>:"Open Config Data.vi"("configuration file path"=w309) -> ("error out"=w304:errorcluster, "refnum"=w305:T6)  [unwired: 8 in, 1 out]
                n152 = call-poly <vilib>:"Read Key.vi"("section"=w303, "error in (no error)"=w304, "key"=w295, "refnum"=w305) -> ("error out"=w299:errorcluster, "value"=w302:string, "refnum out"=w300:T6)  [unwired: 4 in, 1 out]
                n153 = Concatenate Strings(w302, "," ("string"), w296) -> (w297:string)
                n154 = call-poly <vilib>:"Write Key.vi"("section"=w303, "error in (no error)"=w299, "value"=w297, "key"=w295, "refnum"=w300) -> ("error out"=w308:errorcluster, "refnum out"=w307:T6)  [unwired: 4 in, 1 out]
                n155 = property on="FinalizarSolicitud_btn" class="Bool (strict)"("Value"=FALSE) -> ()  [unwired: 2 in, 2 out]
                n156 = property on="SoyCliente_btn" class="Bool (strict)"("Visible"=TRUE) -> ()  [unwired: 2 in, 2 out]
                n157 = call <vilib>:"Close Config Data.vi"("error in (no error)"=w308, "refnum"=w307) -> ()  [unwired: 8 in, 2 out]
                n158 = One Button Dialog(message="Se ha enviado correctamente tu solicitud, esperando aprobacion", button name ("OK")="Aceptar") -> ()  [unwired: 1 out]
              }
              frame #4 {
                n159 = invoke class="VI" method="Default Vals.Reinit All"() -> ()  [unwired: 3 in, 3 out]
              }
            }
            n160 = Bundle By Name(cluster=w206, "Machine"=enum16{"StateMachine", "Queues"}."StateMachine", "States"=T12."goToCreditoPyme") -> (w205:T4)
          }
          frame "CloseApp" {
            n161 = Quit LabVIEW(quit? (T)=TRUE) -> ()
            n162 = Bundle By Name(cluster=w317, "Machine"=enum16{"StateMachine", "Queues"}."StateMachine", "States"=T10."CloseApp") -> (w316:T4)
          }
          frame "goToPersonaMoral" {
            n163 = control-ref of="PersonaFisica_select"() -> (w325:refnum<vi>)
            n164 = control-ref of="PersonaMoral_select"() -> (w326:refnum<vi>)
            n165 = control-ref of="CreditoPyme_select"() -> (w324:refnum<vi>)
            n166 = control-ref of="SolicitudesRecientes_select"() -> (w323:refnum<vi>)
            n167 = call "ControlPageSelected.vi"("PageSelected"=T9."PersonaMoral", "SolicitudesRecientes"=w323, "CreditoPyme"=w324, "PersonaFisica"=w325, "PersonaMoral"=w326) -> ()  [unwired: 7 in]
            n168 = property on="PaginasPrincipales" class="TabCtl (strict)"("Value"=T1."PersonaFisica" ("PaginasPrincipales")) -> ()  [unwired: 2 in, 2 out]
            n169 = property on="MenuPersonaFisica_Moral" class="TabCtl (strict)"("Value"=T11."PersonaMoral1" ("MenuPersonaFisica_Moral")) -> ()  [unwired: 2 in, 2 out]
            n170 = Bundle By Name(cluster=w328, "Machine"=enum16{"StateMachine", "Queues"}."StateMachine", "States"=T10."standBy") -> (w327:T4)
          }
          frame "CheckIsClient" {
            n171 = flat-sequence {
              tunnel: w334 -> [w336]
              tunnel: [w335] -> w331
              tunnel: [w340] -> w332
              tunnel: w333 -> [w339]
              tunnel: w331 -> [w338]
              frame #0 {
                n172 = case shown="True" w336 {
                  tunnel: [_ w337] -> w335
                  frame False {
                  }
                  frame True {
                    n173 = call "PutIDCard.vi"() -> ("ID_CARD"=w337:string)  [unwired: 11 in]
                  }
                }
              }
              frame #1 {
                n174 = Bundle By Name(cluster=w339, "Machine"=enum16{"StateMachine", "Queues"}."StateMachine", "States"=T12."RegisterSolicitudToCheck", "ID_CARD"=w338) -> (w340:T4)
              }
            }
          }
        }
      }
      frame "Queues" {
        n175 = Wait on Notification(notifier=w347, error in (no error)=w346) -> (notification=w345:string)  [unwired: 2 in, 3 out]
        n176 = case shown="\"Moral2_btn\"" w345 {
          tunnel: w344 -> [w351 w355 w358 w364 w369 w373 w380 w384 w388 w394 w398 w402]
          tunnel: [w350 w354 w357 w363 w368 w372 w379 w383 w387 w393 w397 w401] -> w343
          frame "SolicitudesRecientes_btn", Default {
            n177 = Bundle By Name(cluster=w351, "Machine"=enum16{"StateMachine", "Queues"}."StateMachine", "States"=T3."goToSolicitudesRecientes") -> (w350:T4)
          }
          frame "CreditoPyme_btn" {
            n178 = Bundle By Name(cluster=w355, "Machine"=enum16{"StateMachine", "Queues"}."StateMachine", "States"=T3."goToCreditoPyme") -> (w354:T4)
          }
          frame "PersonaFisica_btn" {
            n179 = Bundle By Name(cluster=w358, "Machine"=enum16{"StateMachine", "Queues"}."StateMachine", "States"=T3."goToPersonaFisica", "TipoPersona"="FISICA") -> (w357:T4)
          }
          frame "PersonaMoral_btn" {
            n180 = Bundle By Name(cluster=w364, "Machine"=enum16{"StateMachine", "Queues"}."StateMachine", "States"=T10."goToPersonaMoral", "TipoPersona"="MORAL") -> (w363:T4)
          }
          frame "CloseApp" {
            n181 = Bundle By Name(cluster=w369, "Machine"=enum16{"StateMachine", "Queues"}."StateMachine", "States"=T10."CloseApp") -> (w368:T4)
          }
          frame "SoyCliente_btn" {
            n182 = Bundle By Name(cluster=w373, "Machine"=enum16{"StateMachine", "Queues"}."StateMachine", "States"=T10."goToPersonaFisica", "TipoPersona"="FISICA", "EsCliente?"=TRUE) -> (w372:T4)
          }
          frame "Moral1_btn" {
            n183 = Bundle By Name(cluster=w380, "Machine"=enum16{"StateMachine", "Queues"}."StateMachine", "States"=T10."goToPersonaMoral1", "TipoPersona"="MORAL") -> (w379:T4)
          }
          frame "IrADatosEspecificos_btn" {
            n184 = Bundle By Name(cluster=w384, "Machine"=enum16{"StateMachine", "Queues"}."StateMachine", "States"=T10."goToDatosEspecificos") -> (w383:T4)
          }
          frame "FinalizarSolicitud_btn" {
            n185 = Bundle By Name(cluster=w388, "Machine"=enum16{"StateMachine", "Queues"}."StateMachine", "States"=T12."CheckIsClient") -> (w387:T4)
          }
          frame "NoTengoCuenta_btn" {
            n186 = Bundle By Name(cluster=w394, "Machine"=enum16{"StateMachine", "Queues"}."StateMachine", "States"=T12."goToPersonaFisica", "EsCliente?"=FALSE, "TipoPersona"="FISICA") -> (w393:T4)
          }
          frame "Moral2_btn" {
            n187 = Bundle By Name(cluster=w398, "Machine"=enum16{"StateMachine", "Queues"}."StateMachine", "States"=T10."goToPersonaMoral2") -> (w397:T4)
          }
          frame "inicio_btn" {
            n188 = Bundle By Name(cluster=w402, "Machine"=enum16{"StateMachine", "Queues"}."StateMachine", "States"=T10."goToCreditoPyme") -> (w401:T4)
          }
        }
      }
    }
  }
  n189 = while {
    shift-right: [w404] -> _
    shift-left: w16 -> [w406]
    shift-right: [w403] -> _
    shift-left: w15 -> [w405]
    stop <- w403 stop-if-true
    n190 = event shown="[8] \"SoyCliente_btn\": Value Change" {
      selector: _ -> [_ _ _ _ _ _ _ _ _ _ _ _ _]
      dyn-events: _ -> [_ _ _ _ _ _ _ _ _ _ _ _ _]
      timeout: _ -> [_ _ _ _ _ _ _ _ _ _ _ _ _]
      tunnel: w406 -> [w407 w414 w420 w426 w432 w438 w444 w449 w456 w461 w467 w473 w478]
      tunnel: w405 -> [w408 w413 w419 w425 w431 w437 w443 w448 w455 w460 w466 w472 w477]
      tunnel: [w408 w412 w418 w424 w430 w436 w441 w447 w453 w459 w465 w471 w476] -> w403
      tunnel: [w407 w411 w417 w423 w429 w435 w442 w446 w454 w458 w464 w470 w475] -> w404
      event Timeout {
        n191 = event-data() -> ()  [unwired: 1 in, 1 out]
      }
      event "CreditoPyme_btn": Value Change {
        n192 = event-data() -> ()  [unwired: 1 in, 1 out]
        n193 = Send Notification(notification="CreditoPyme_btn", notifier=w414, error in (no error)=w413) -> (notifier out=w411:refnum<notifier>, error out=w412:errorcluster)
        n194 = property on="CreditoPyme_btn" class="Bool (strict)"("Value"=FALSE ("CreditoPyme_btn")) -> ()  [unwired: 2 in, 2 out]
      }
      event "SolicitudesRecientes_btn": Value Change {
        n195 = event-data() -> ()  [unwired: 1 in, 1 out]
        n196 = Send Notification(notification="SolicitudesRecientes_btn", notifier=w420, error in (no error)=w419) -> (notifier out=w417:refnum<notifier>, error out=w418:errorcluster)
        n197 = property on="SolicitudesRecientes_btn" class="Bool (strict)"("Value"=FALSE ("SolicitudesRecientes_btn")) -> ()  [unwired: 2 in, 2 out]
      }
      event "PersonaFisica_btn": Value Change {
        n198 = event-data() -> ()  [unwired: 1 in, 1 out]
        n199 = Send Notification(notification="PersonaFisica_btn", notifier=w426, error in (no error)=w425) -> (notifier out=w423:refnum<notifier>, error out=w424:errorcluster)
        n200 = property on="PersonaFisica_btn" class="Bool (strict)"("Value"=FALSE ("PersonaFisica_btn")) -> ()  [unwired: 2 in, 2 out]
      }
      event "PersonaMoral_btn": Value Change {
        n201 = event-data() -> ()  [unwired: 1 in, 1 out]
        n202 = Send Notification(notification="PersonaMoral_btn", notifier=w432, error in (no error)=w431) -> (notifier out=w429:refnum<notifier>, error out=w430:errorcluster)
        n203 = property on="PersonaMoral_btn" class="Bool (strict)"("Value"=FALSE ("PersonaMoral_btn")) -> ()  [unwired: 2 in, 2 out]
      }
      event "Moral1_btn": Value Change {
        n204 = event-data() -> ()  [unwired: 1 in, 1 out]
        n205 = Send Notification(notification="Moral1_btn", notifier=w438, error in (no error)=w437) -> (notifier out=w435:refnum<notifier>, error out=w436:errorcluster)
        n206 = property on="Moral1_btn" class="Bool (strict)"("Value"=FALSE ("Moral1_btn")) -> ()  [unwired: 2 in, 2 out]
      }
      event "Moral2_btn": Value Change {
        n207 = event-data() -> ()  [unwired: 1 in, 1 out]
        n208 = Send Notification(notification="Moral2_btn", notifier=w444, error in (no error)=w443) -> (notifier out=w442:refnum<notifier>, error out=w441:errorcluster)
        n209 = property on="Moral2_btn" class="Bool (strict)"("Value"=FALSE ("Moral2_btn")) -> ()  [unwired: 2 in, 2 out]
      }
      event Panel Close? {
        n210 = event-data() -> ()  [unwired: 1 in, 1 out]
        n211 = Send Notification(notification="CloseApp", notifier=w449, error in (no error)=w448) -> (notifier out=w446:refnum<notifier>, error out=w447:errorcluster)
        n212 = event-data("Discard?"=TRUE) -> ()  [unwired: 1 in, 1 out]
      }
      event "SoyCliente_btn": Value Change {
        n213 = event-data() -> ()  [unwired: 1 in, 1 out]
        n214 = Send Notification(notification="SoyCliente_btn", notifier=w456, error in (no error)=w455) -> (notifier out=w454:refnum<notifier>, error out=w453:errorcluster)
        n215 = property on="SoyCliente_btn" class="Bool (strict)"("Value"=FALSE ("SoyCliente_btn")) -> ()  [unwired: 2 in, 2 out]
      }
      event "NoTengoCuenta_btn": Value Change {
        n216 = event-data() -> ()  [unwired: 1 in, 1 out]
        n217 = Send Notification(notification="NoTengoCuenta_btn", notifier=w461, error in (no error)=w460) -> (notifier out=w458:refnum<notifier>, error out=w459:errorcluster)
      }
      event "IrADatosEspecificos_btn": Value Change {
        n218 = event-data() -> ()  [unwired: 1 in, 1 out]
        n219 = Send Notification(notification="IrADatosEspecificos_btn", notifier=w467, error in (no error)=w466) -> (notifier out=w464:refnum<notifier>, error out=w465:errorcluster)
        n220 = property on="IrADatosEspecificos_btn" class="Bool (strict)"("Value"=FALSE ("IrASolicitud_btn")) -> ()  [unwired: 2 in, 2 out]
      }
      event "inicio_btn": Value Change {
        n221 = event-data() -> ()  [unwired: 1 in, 1 out]
        n222 = Send Notification(notification="inicio_btn", notifier=w473, error in (no error)=w472) -> (notifier out=w470:refnum<notifier>, error out=w471:errorcluster)
        n223 = property on="inicio_btn" class="Bool (strict)"("Value"=FALSE ("inicio_btn")) -> ()  [unwired: 2 in, 2 out]
      }
      event "FinalizarSolicitud_btn": Value Change {
        n224 = event-data() -> ()  [unwired: 1 in, 1 out]
        n225 = Send Notification(notification="FinalizarSolicitud_btn", notifier=w478, error in (no error)=w477) -> (notifier out=w475:refnum<notifier>, error out=w476:errorcluster)
      }
    }
  }
  n226 = call <vilib>:"Close Config Data.vi"("error in (no error)"=w2, "refnum"=w3) -> ()  [unwired: 8 in, 2 out]
